vi "get_base_frequency.vi"(8 "error in (no error)":errorcluster, 11 "FPGAWrapperAK101022Resonance in":refnum<class "FPGAWrapperAK101022Resonance.lvclass">) -> (0 "error out":errorcluster, 2 "base frequency":dbl[unit]=40000000.0, 3 "FPGAWrapperAK101022Resonance out":refnum<class "FPGAWrapperAK101022Resonance.lvclass">)   [LabVIEW 2010, in "FPGAWrapperAK101022Resonance.lvclass"]
uses:
  FPGAWrapperAK101022Resonance.lvclass
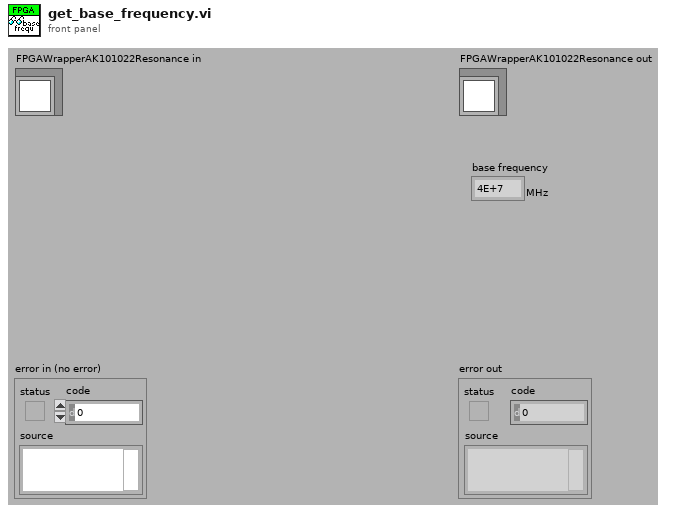
[diagram p1: front panel]
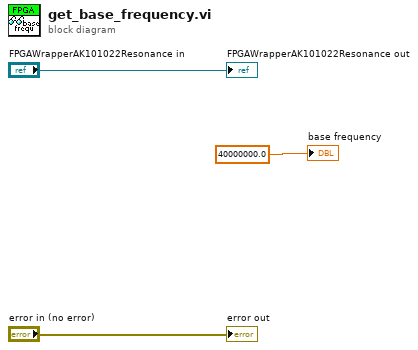
[diagram p0: block diagram]
diagram:
  "error out" <- "error in (no error)"
  "FPGAWrapperAK101022Resonance out" <- "FPGAWrapperAK101022Resonance in"
  "base frequency" <- dbl[unit] 40000000.0 ("base frequency")
